vi "VS JKI.vi"() -> ()   [LabVIEW 2016, in "LVJSON Tests.lvlib"]
uses:
  LVJSON Tests.lvlib
  <vilib>/National Instruments/JSON Support for LabVIEW/JSON Data Classes/JSON Numeric/JSON Numeric.lvclass
  C:/Program Files (x86)/National Instruments/LabVIEW 2016/vi.lib/National Instruments/JSON Support for LabVIEW/JSON Data Classes/JSON Datatype/JSON Null.lvclass
  <vilib>/National Instruments/JSON Support for LabVIEW/JSON Data Classes/JSON Helper/Parsing/Parse Value.vi
  <vilib>/National Instruments/JSON Support for LabVIEW/JSON Data Classes/JSON Object/New JSON Object (Multi).vi
  <vilib>/National Instruments/JSON Support for LabVIEW/JSON Data Classes/JSON Numeric/New JSON Numeric.vi
  <vilib>/rajsite/i3-json/JSON Generation/Add Object Parameter Files/Add Object Parameter - Numeric.vi
  <vilib>/rajsite/i3-json/JSON Generation/Create Value Files/Create Value - Object.vi
  <vilib>/National Instruments/JSON Support for LabVIEW/JSON Data Classes/JSON Datatype/JSON Null.lvclass
  <vilib>/National Instruments/JSON Support for LabVIEW/JSON Data Classes/JSON Object/JSON Object.lvclass
  <vilib>/National Instruments/JSON Support for LabVIEW/JSON Data Classes/JSON Helper/JSON Helper.lvclass
  <vilib>/rajsite/i3-json/i3-json.lvlib
  C:/Program Files (x86)/National Instruments/LabVIEW 2016/vi.lib/National Instruments/JSON Support for LabVIEW/JSON Data Classes/JSON Basic Type/JSON Literal.lvclass
panel:
  out "lvjson generation faster?":bool
  out "generation ratio":dbl
  out "lvjson generation time":dbl
  out "i3 generation time":dbl
  out "unflatten ratio":dbl
  out "flatten ratio":dbl
  in  "# of elements":i32
  out "lvjson flatten faster?":bool
  out "lvjson unflatten faster?":bool
  out "i3 String":string
  out "lvjson String":string
  out "lvjson unflatten time":dbl
  out "lvjson flatten time":dbl
  out "i3 unflatten time":dbl
  out "i3 flatten time":dbl
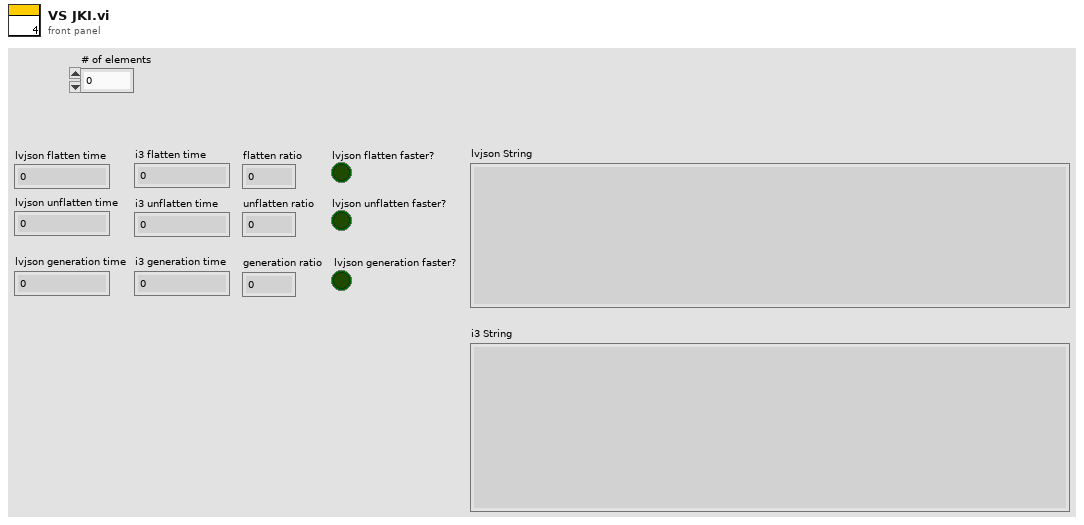
[diagram p1: front panel]
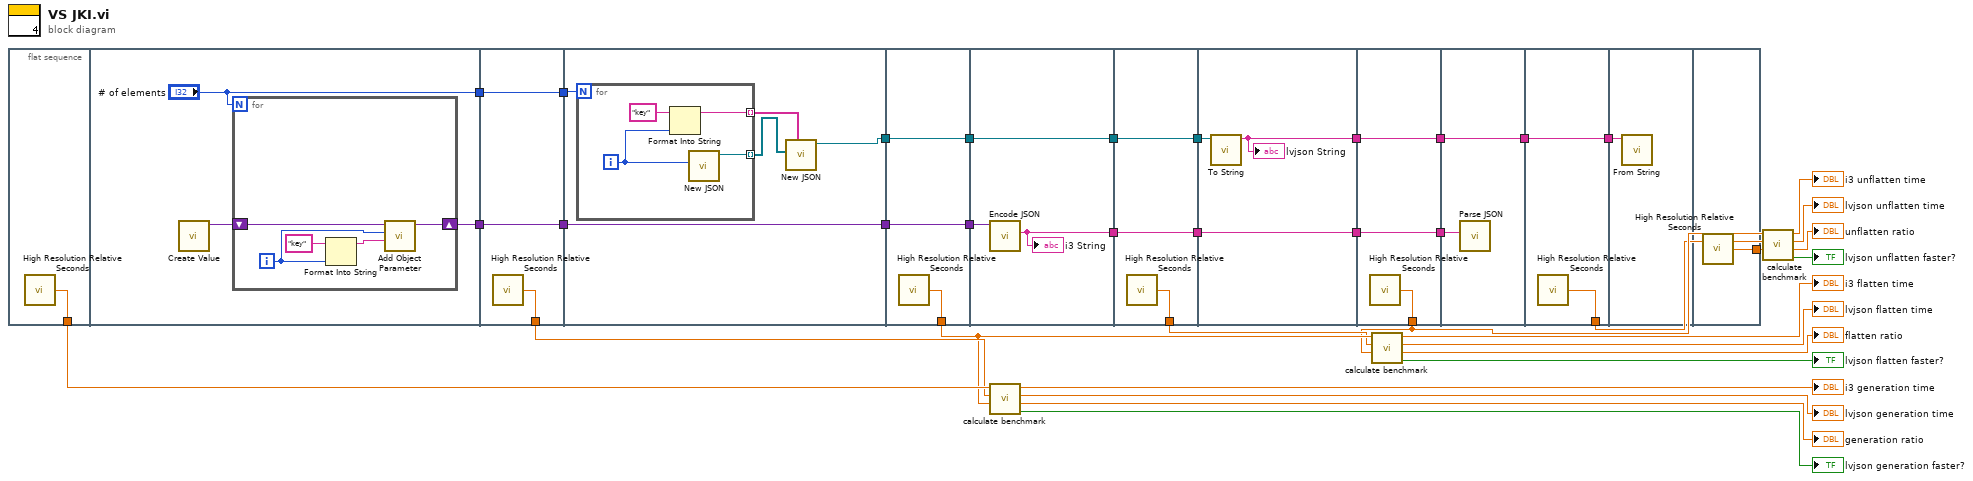
[diagram p0: block diagram]
diagram:
  n1 = flat-sequence {
    tunnel: [w38] -> w8
    tunnel: ["# of elements"] -> w29
    tunnel: [w39] -> w27
    tunnel: w29 -> [w49]
    tunnel: [w49] -> w28
    tunnel: w27 -> [w47]
    tunnel: [w48] -> w7
    tunnel: [w47] -> w23
    tunnel: w28 -> [w54]
    tunnel: w23 -> [w53]
    tunnel: [w53] -> w12
    tunnel: [w50] -> w10
    tunnel: w12 -> [w61]
    tunnel: [w61] -> w11
    tunnel: w10 -> [w60]
    tunnel: [w60] -> w9
    tunnel: [w59] -> w6
    tunnel: w11 -> [w64]
    tunnel: w9 -> [w63]
    tunnel: [w63] -> w22
    tunnel: [w62] -> w20
    tunnel: [w67] -> w5
    tunnel: w22 -> [w66]
    tunnel: [w66] -> w21
    tunnel: w20 -> [w65]
    tunnel: [w65] -> w19
    tunnel: w21 -> [w70]
    tunnel: w19 -> [w69]
    tunnel: [w69] -> w18
    tunnel: [w68] -> w16
    tunnel: [w73] -> w4
    tunnel: w18 -> [w72]
    tunnel: [w72] -> w17
    tunnel: w16 -> [w71]
    tunnel: [w71] -> w15
    tunnel: w17 -> [w75]
    tunnel: w15 -> [w74]
    tunnel: [w74] -> w14
    tunnel: [w77] -> w3
    tunnel: w14 -> [w76]
    tunnel: [w76] -> w13
    tunnel: w13 -> [w78]
    tunnel: [w79] -> w2
    frame #0 {
      n2 = call <vilib>:"High Resolution Relative Seconds.vi"() -> ("relative seconds"=w38:dbl)
    }
    frame #1 {
      n3 = call-poly <vilib>:"Create Value.vi"() -> ("JSON Tree"=w41:variant)  [unwired: 10 in, 1 out]
      n4 = for {
        N: "# of elements" -> [_]
        shift-right: [w42] -> w39
        shift-left: w41 -> [w46]
        i -> [w43]
        n5 = Format Into String(initial string="key", w43) -> (resulting string=w44:string)  [unwired: 2 in, 1 out]
        n6 = call-poly <vilib>:"Add Object Parameter.vi"("Name"=w44, "Numeric"=w43, "JSON Tree in (JSON Object)"=w46) -> ("JSON Tree out (JSON Object)"=w42:variant)  [unwired: 7 in, 1 out]
      }
    }
    frame #2 {
      n7 = call <vilib>:"High Resolution Relative Seconds.vi"() -> ("relative seconds"=w48:dbl)
    }
    frame #3 {
      n8 = for {
        N: w54 -> [_]
        tunnel: [w57] -> w51 mode=indexing
        tunnel: [w55] -> w52 mode=indexing
        i -> [w56]
        n9 = Format Into String(initial string="key", w56) -> (resulting string=w57:string)  [unwired: 2 in, 1 out]
        n10 = call-poly <vilib>:"New JSON.vi"("value"=w56) -> ("JSON String out"=w55:refnum<class "JSON Numeric.lvclass">)  [unwired: 9 in, 1 out]
      }
      n11 = call-poly <vilib>:"New JSON.vi"("keys"=w51, "values"=w52) -> ("JSON Object out"=w50:refnum<class "JSON Object.lvclass">)  [unwired: 8 in, 1 out]
    }
    frame #4 {
      n12 = call <vilib>:"High Resolution Relative Seconds.vi"() -> ("relative seconds"=w59:dbl)
    }
    frame #5 {
      n13 = call <vilib>:"Encode JSON.vi"("JSON Tree In"=w64) -> ("String"=w62:string)  [unwired: 5 in, 1 out]
      "i3 String" <- w62
    }
    frame #6 {
      n14 = call <vilib>:"High Resolution Relative Seconds.vi"() -> ("relative seconds"=w67:dbl)
    }
    frame #7 {
      n15 = call-dynamic "To String.vi"("JSON Object in"=w70) -> ("String"=w68:string)  [unwired: 9 in, 1 out]
      "lvjson String" <- w68
    }
    frame #8 {
      n16 = call <vilib>:"High Resolution Relative Seconds.vi"() -> ("relative seconds"=w73:dbl)
    }
    frame #9 {
      n17 = call <vilib>:"Parse JSON.vi"("JSON String"=w75) -> ()  [unwired: 7 in, 4 out]
    }
    frame #10 {
      n18 = call <vilib>:"High Resolution Relative Seconds.vi"() -> ("relative seconds"=w77:dbl)
    }
    frame #11 {
      n19 = call <vilib>:"From String.vi"("JSON String"=w78) -> ()  [unwired: 9 in, 2 out]
    }
    frame #12 {
      n20 = call <vilib>:"High Resolution Relative Seconds.vi"() -> ("relative seconds"=w79:dbl)
    }
  }
  n21 = call "calculate benchmark.vi"("end"=w6, "middle"=w7, "beginning"=w8) -> ("lvjson faster?"=→"lvjson generation faster?":bool, "ratio"=→"generation ratio":dbl, "lvjson time"=→"lvjson generation time":dbl, "i3 time"=→"i3 generation time":dbl)  [unwired: 5 in]
  n22 = call "calculate benchmark.vi"("end"=w4, "middle"=w5, "beginning"=w6) -> ("lvjson faster?"=→"lvjson flatten faster?":bool, "ratio"=→"flatten ratio":dbl, "lvjson time"=→"lvjson flatten time":dbl, "i3 time"=→"i3 flatten time":dbl)  [unwired: 5 in]
  n23 = call "calculate benchmark.vi"("end"=w2, "middle"=w3, "beginning"=w4) -> ("lvjson faster?"=→"lvjson unflatten faster?":bool, "ratio"=→"unflatten ratio":dbl, "lvjson time"=→"lvjson unflatten time":dbl, "i3 time"=→"i3 unflatten time":dbl)  [unwired: 5 in]
